vi "Create (String).vi"(7 "Options":T1, 8 "error in (no error)":errorcluster, 10 "Base URL (None)":string, 11 "Input Pattern":string) -> (0 "error out":errorcluster, 3 "URLPattern out":refnum<class "URLPattern.lvclass">)   [LabVIEW 2020, in "Stream.lvlib" / "URLPattern.lvclass"]
uses:
  URLPattern.lvclass
  Options.ctl
  URLPattern.lvclass/URLPattern.ctl
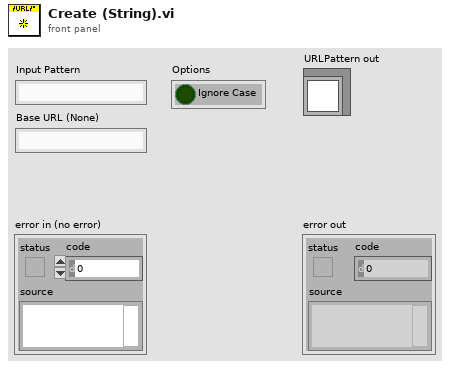
[diagram p1: front panel]
types:
  T1 = typedef "Stream.lvlib/URLPattern.lvclass/Options.ctl" = cluster{"Ignore Case":bool}
  T2 = typedef "Stream.lvlib/URLPattern.lvclass/URL Pattern Init.ctl" = cluster{"protocol":string, "username":string, "password":string, "hostname":string, "port":string, "pathname":string, "search":string, "hash":string}
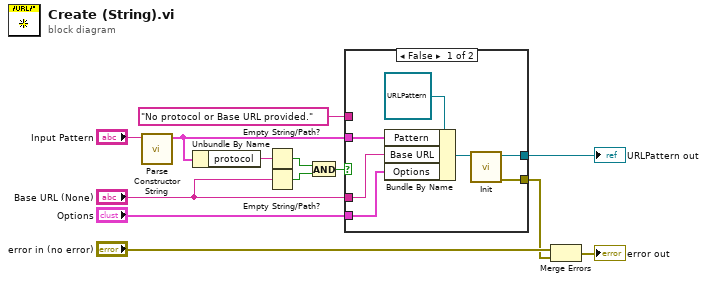
[diagram p0: block diagram]
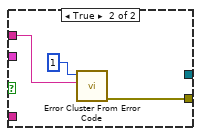
[diagram p2: hidden frame]
diagram:
  n1 = call "Parse Constructor String.vi"("Input"="Input Pattern") -> ("Result"=w10:T2)  [unwired: 9 in, 1 out]
  n2 = Unbundle By Name(w10) -> ("protocol"=w9:string)
  n3 = Empty String/Path?(string/path=w9) -> (empty?=w8:bool)
  n4 = Empty String/Path?(string/path="Base URL (None)") -> (empty?=w7:bool)
  n5 = And(x=w8, y=w7) -> (x .and. y?=w6:bool)
  n6 = case shown="False" w6 {
    tunnel: [w15 _] -> w11
    tunnel: w10 -> [w19 _]
    tunnel: "Base URL (None)" -> [w18 _]
    tunnel: [w14 w22] -> w3
    tunnel: "Options" -> [w17 _]
    tunnel: "No protocol or Base URL provided." ("error message (\"\")") -> [_ w21]
    frame False {
      n7 = Bundle By Name(cluster=refnum<class "URLPattern.lvclass"> refnum ("URLPattern in"), "Pattern"=w19, "Base URL"=w18, "Options"=w17) -> (w16:refnum<class "URLPattern.lvclass">)
      n8 = call "Init.vi"("URLPattern in"=w16) -> ("error out"=w14:errorcluster, "URLPattern out"=w15:refnum<class "URLPattern.lvclass">)  [unwired: 9 in]
    }
    frame True {
      n9 = call <vilib>:"Error Cluster From Error Code.vi"("error message (\"\")"=w21, "error code (0)"=1) -> ("error out"=w22:errorcluster)  [unwired: 7 in]
    }
  }
  "URLPattern out" <- w11
  n10 = Merge Errors("error in (no error)", w3) -> (→"error out":errorcluster)
